vi "Init SPI CS.vi"(7 "CS GPIO":T1=5, 8 "error in (no error)":errorcluster, 10 "CS Active Low (T)":bool=TRUE, 11 "VisaSession in":refnum<class "VisaSession.lvclass">) -> (0 "error out":errorcluster, 2 "SPI CS":refnum<class "SPI CS.lvclass">, 3 "VisaSession out":refnum<class "VisaSession.lvclass">)   [LabVIEW 2020, in "CTI.lvlib" / "VisaSession.lvclass"]
uses:
  VisaSession.lvclass
  VisaSession.lvclass/VisaSession.ctl
  Session/Session.lvclass
  SPI CS/SPI CS.lvclass
  GPIO Number.ctl
  CTI.lvlib
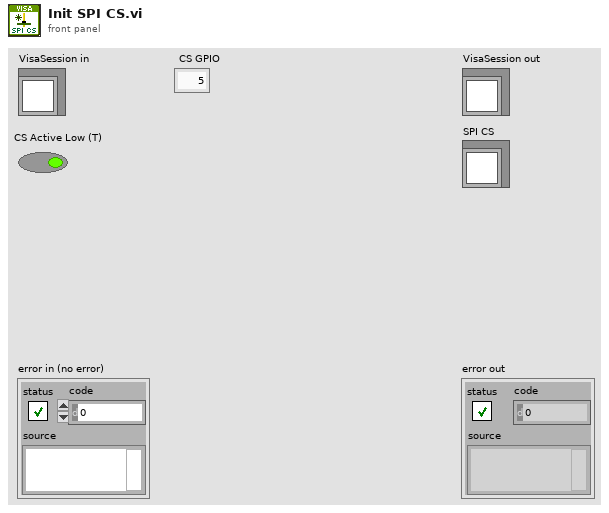
[diagram p1: front panel]
types:
  T1 = typedef "CTI.lvlib/GPIO Number.ctl" = i8
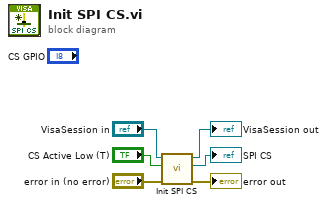
[diagram p0: block diagram]
diagram:
  n1 = call-parent "Init SPI CS.vi"("error in (no error)"="error in (no error)", "CS Active Low (T)"="CS Active Low (T)", "Session in"="VisaSession in") -> ("error out"=→"error out":errorcluster, "SPI CS"=→"SPI CS":refnum<class "SPI CS.lvclass">, "Session out"=→"VisaSession out":refnum<class "VisaSession.lvclass">)  [unwired: 6 in]
